vi "Secure SSL Client Test.vi"() -> ()   [LabVIEW 2013]
uses:
  SSL_Lib/SSL-Lib/Library Paths.ctl
  SSL_Lib/SSL-Context/SSL Verify Mode.ctl
  SSL_Lib/SSL-Context/SSL Options.ctl
  SSL Client Context/SSL Client Context.lvclass/SSL Client Context.ctl
  SSL Client Context/SSL Client Context.lvclass
  SSL Client Socket/SSL Client Socket.lvclass
  <vilib>/MediaMongrels Ltd/WebSockets/WebSockets/WebSocket Client/WebSocket Client.lvclass
  <vilib>/MediaMongrels Ltd/WebSockets/WebSockets/WebSocket/WebSocket.lvclass/WebSocket.ctl
  SSL Client Context/Write Verification Options.vi
  SSL Client Context/Write Verification CA Bundle Path.vi
  SSL Client Context/Write SSL Options.vi
  SSL Client Context/Write Cipher List.vi
  <vilib>/MediaMongrels Ltd/WebSockets/WebSockets/WebSocket/Read Return Headers.vi
  SSL_Lib/SSL-Lib/SSL-Lib.lvclass
  SSL_Lib/SSL-Context/SSL-Context.lvclass
panel:
  out "Return Headers 2":variant
  out "Data 2":string
  out "Data":string
  out "Return Headers":variant
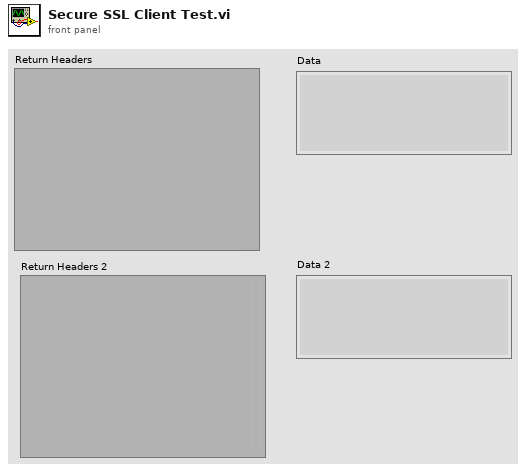
[diagram p1: front panel]
types:
  T1 = typedef "SSL_Lib.lvlib/SSL-Context.lvclass/SSL Options.ctl" = i32
  T2 = typedef "SSL_Lib.lvlib/SSL-Context.lvclass/SSL Verify Mode.ctl" = i32
  T3 = typedef "SSL_Lib.lvlib/SSL-Lib.lvclass/Library Paths.ctl" = cluster{"SSL Library Path":path, "Crypto Library Path":path}
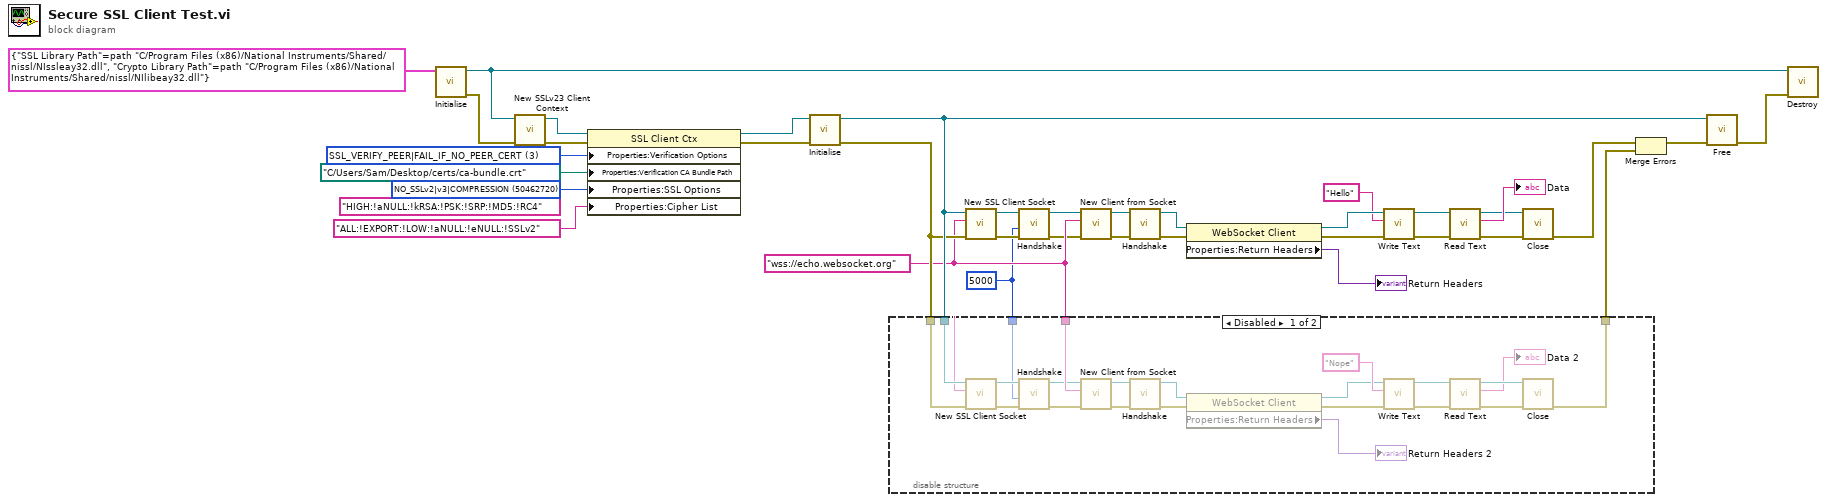
[diagram p0: block diagram]
diagram:
  w1 = u32 5000 ("Timeout (5000ms)")
  (unwired) "HIGH:!aNULL:!kRSA:!PSK:!SRP:!MD5:!RC4" ("Cipher List")
  w12 = T1 50462720 items=["None"=0, "NO_SSLv2|v3|COMPRESSION"=50462720, "SSL_OP_NO_COMPRESSION"=131072, "SSL_OP_NO_SSLv2"=16777216, "SSL_OP_NO_SSLv3"=33554432, "SSL_OP_NO_TLSv1"=67108864, "SSL_OP_NO_TLSv1_2"=134217728, "SSL_OP_NO_TLSv1_1"=268435456] ("SSL Options")
  w14 = T2 3 items=["SSL_VERIFY_PEER|FAIL_IF_NO_PEER_CERT"=3, "SSL_VERIFY_NONE"=0, "SSL_VERIFY_PEER"=1, "SSL_VERIFY_FAIL_IF_NO_PEER_CERT"=2, "SSL_VERIFY_CLIENT_ONCE"=4] ("Verification Options")
  w7 = "wss://echo.websocket.org" ("WebSocket URL")
  n1 = call "Initialise.vi"("Library Paths"=T3 {"SSL Library Path"=path "C:/Program Files (x86)/National Instruments/Shared/nissl/NIssleay32.dll", "Crypto Library Path"=path "C:/Program Files (x86)/National Instruments/Shared/nissl/NIlibeay32.dll"}) -> ("error out"=w22:errorcluster, "SSL-Lib out"=w20:refnum<class "SSL-Lib.lvclass">)  [unwired: 9 in]
  n2 = call "New SSLv23 Client Context.vi"("error in (no error)"=w22, "SSL-Lib"=w20) -> ("error out"=w21:errorcluster, "SSL Client Context out"=w16:refnum<class "SSL Client Context.lvclass">)  [unwired: 8 in]
  n3 = property class="SSL Client Ctx"(reference=w16, error in=w21, "Properties:Verification Options"=w14, "Properties:Verification CA Bundle Path"=path "C:/Users/Sam/Desktop/certs/ca-bundle.crt" ("Path to CA bundle"), "Properties:SSL Options"=w12, "Properties:Cipher List"="ALL:!EXPORT:!LOW:!aNULL:!eNULL:!SSLv2" ("Cipher List")) -> (reference out=w15:refnum<class "SSL Client Context.lvclass">, error out=w17:errorcluster)
  n4 = call-dynamic "Initialise.vi"("error in (no error)"=w17, "OpenSSL Client Context in"=w15) -> ("error out"=w8:errorcluster, "OpenSSL Client Context out"=w9:refnum<class "SSL Client Context.lvclass">)  [unwired: 8 in]
  n5 = disable-structure shown="Disabled" {
    disable-tunnel: w9 -> [w44 _]
    disable-tunnel: w8 -> [w43 _]
    disable-tunnel: w7 -> [w42 _]
    disable-tunnel: [w41 _] -> w5
    disable-tunnel: w1 -> [w37 _]
    frame Disabled {
      n6 = call "New SSL Client Socket.vi"("error in (no error)"=w43, "Hostname / URL"=w42, "SSL Client Ctx"=w44) -> ("error out"=w39:errorcluster, "SSL Client Skt out"=w58:refnum<class "SSL Client Socket.lvclass">)  [unwired: 7 in]
      n7 = call-dynamic "Handshake.vi"("error in (no error)"=w39, "Timeout (5000ms)"=w37, "OpenSSL in"=w58) -> ("error out"=w38:errorcluster, "OpenSSL out"=w40:refnum<class "SSL Client Socket.lvclass">)  [unwired: 7 in]
      n8 = call <vilib>:"New Client from Socket.vi"("error in (no error)"=w38, "WebSocket URL"=w42, "Socket in"=w40) -> ("error out"=w45:errorcluster, "WebSocket Client out"=w46:refnum<class "WebSocket Client.lvclass">)  [unwired: 7 in]
      n9 = call-dynamic "Handshake.vi"("error in (no error)"=w45, "WebSocket Client in"=w46) -> ("error out"=w47:errorcluster, "WebSocket Client out"=w48:refnum<class "WebSocket Client.lvclass">)  [unwired: 8 in]
      n10 = property class="WebSocket Client"(reference=w48, error in=w47) -> (reference out=w51:refnum<class "WebSocket Client.lvclass">, error out=w50:errorcluster, "Properties:Return Headers"=→"Return Headers 2":variant)
      n11 = call-dynamic "Write Text.vi"("error in (no error)"=w50, "String Data"="Nope", "WebSocket in"=w51) -> ("error out"=w53:errorcluster, "WebSocket out"=w54:refnum<class "WebSocket Client.lvclass">)  [unwired: 7 in]
      n12 = call-dynamic "Read Text.vi"("error in (no error)"=w53, "WebSocket in"=w54) -> ("error out"=w56:errorcluster, "Data"=→"Data 2":string, "WebSocket out"=w57:refnum<class "WebSocket Client.lvclass">)  [unwired: 7 in]
      n13 = call-dynamic "Close.vi"("error in (no error)"=w56, "WebSocket in"=w57) -> ("error out"=w41:errorcluster)  [unwired: 9 in]
    }
    frame Enabled {
    }
  }
  n14 = call "New SSL Client Socket.vi"("error in (no error)"=w8, "Hostname / URL"=w7, "SSL Client Ctx"=w9) -> ("error out"=w3:errorcluster, "SSL Client Skt out"=w10:refnum<class "SSL Client Socket.lvclass">)  [unwired: 7 in]
  n15 = call-dynamic "Handshake.vi"("error in (no error)"=w3, "Timeout (5000ms)"=w1, "OpenSSL in"=w10) -> ("error out"=w2:errorcluster, "OpenSSL out"=w4:refnum<class "SSL Client Socket.lvclass">)  [unwired: 7 in]
  n16 = call <vilib>:"New Client from Socket.vi"("error in (no error)"=w2, "WebSocket URL"=w7, "Socket in"=w4) -> ("error out"=w36:errorcluster, "WebSocket Client out"=w35:refnum<class "WebSocket Client.lvclass">)  [unwired: 7 in]
  n17 = call-dynamic "Handshake.vi"("error in (no error)"=w36, "WebSocket Client in"=w35) -> ("error out"=w34:errorcluster, "WebSocket Client out"=w33:refnum<class "WebSocket Client.lvclass">)  [unwired: 8 in]
  n18 = property class="WebSocket Client"(reference=w33, error in=w34) -> (reference out=w30:refnum<class "WebSocket Client.lvclass">, error out=w31:errorcluster, "Properties:Return Headers"=→"Return Headers":variant)
  n19 = call-dynamic "Write Text.vi"("error in (no error)"=w31, "String Data"="Hello", "WebSocket in"=w30) -> ("error out"=w28:errorcluster, "WebSocket out"=w27:refnum<class "WebSocket Client.lvclass">)  [unwired: 7 in]
  n20 = call-dynamic "Read Text.vi"("error in (no error)"=w28, "WebSocket in"=w27) -> ("error out"=w25:errorcluster, "Data"=→"Data":string, "WebSocket out"=w24:refnum<class "WebSocket Client.lvclass">)  [unwired: 7 in]
  n21 = call-dynamic "Close.vi"("error in (no error)"=w25, "WebSocket in"=w24) -> ("error out"=w18:errorcluster)  [unwired: 9 in]
  n22 = Merge Errors(w18, w5) -> (w6:errorcluster)
  n23 = call-dynamic "Free.vi"("error in (no error)"=w6, "OpenSSL Context in"=w9) -> ("error out"=w19:errorcluster)  [unwired: 9 in]
  n24 = call "Destroy.vi"("error in (no error)"=w19, "SSL-Lib in"=w20) -> ()  [unwired: 9 in, 1 out]
